vi "Begin.vi"(8 "error in":errorcluster) -> (0 "error out":errorcluster)   [LabVIEW 2023]
doc: "Called before other user functions, this VI is expected to open initial I/O refnums, load in file data, and do all program initialization. Notice that the <B>error out</B> terminal is simply used for data flow. Wiring it to other structures or subVIs ensures that this VI runs first."
uses:
  <vilib>/Rock Robotics/WPI/DriverStation/WPI_DriverStationRobotMode2.ctl
  <vilib>/Rock Robotics/WPI/Joystick/WPI_JoystickDeviceEnum.ctl
  <vilib>/Rock Robotics/WPI/SafetyOutput/WPI_SafetyOutputConfigMenu.ctl
  Robot Global Data.vi
  <vilib>/Rock Robotics/Network Tables/NT Write String Array.vi
  <vilib>/Rock Robotics/WPI/RobotDrive/WPI_RobotDriveOpen2MotorWithExistingMotors.vi
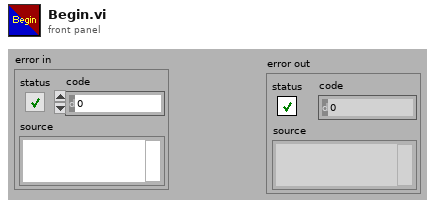
[diagram p1: front panel]
types:
  T1 = typedef "WPI_SafetyOutputConfigMenu.ctl" = enum16{"Enable", "Disable"}
  T2 = typedef "WPI_JoystickDeviceEnum.ctl" = enum16{"USB 0", "USB 1", "USB 2", "USB 3", "USB 4", "USB 5"}
  T3 = typedef "WPI_DriverStationRobotMode2.ctl" = enum16{"Autonomous Disabled", "Autonomous Enabled", "Teleop Disabled", "Teleop Enabled", "Disconnected", "Finish", "Test Disabled", "Test Enabled", "Emergency Stopped"}
  T4 = typedef "WPI_MotorControlDeviceRef.ctl" = cluster{"DeviceStatus":errorcluster, "Type":T5, "PWM":cluster{"PWM Channel":T6, "DeadBand":T7}, "CAN":cluster{"Device Number":u8, "SetOutput VI Ref":variant, "GetOutput VI Ref":variant, "Enable VI Ref":variant, "Disable VI Ref":variant, "Data":variant}, "Invert":bool, "DIO PWM":cluster{"PWM \"Enable\" Channel":T6, "DIOChannel":T8, "PWM Rate":dbl}}
  T5 = typedef "WPI_MotorControlType.ctl" = enum16{"PWM", "CAN", "DIO PWM"}
  T6 = typedef "FPGA_DIOPWMChannel.ctl" = enum8{"PWM 0", "PWM 1", "PWM 2", "PWM 3", "PWM 4", "PWM 5", "PWM 6", "PWM 7", "PWM 8", "PWM 9", "PWM MXP 0", "PWM MXP 1", "PWM MXP 2", "PWM MXP 3", "PWM MXP 4", "PWM MXP 5", "PWM MXP 6", "PWM MXP 7", "PWM MXP 8", "PWM MXP 9", "Invalid"}
  T7 = typedef "WPI_PWMDeadband.ctl" = cluster{"Name":string, "maxPositivePwm":i32, "minPositivePwm":i32, "centerPwm":i32, "maxNegativePwm":i32, "minNegativePwm":i32, "angularRange":u16}
  T8 = typedef "FPGA_DIOChannel.ctl" = enum8{"DIO 0", "DIO 1", "DIO 2", "DIO 3", "DIO 4", "DIO 5", "DIO 6", "DIO 7", "DIO 8", "DIO 9", "DIO MXP 0", "DIO MXP 1", "DIO MXP 2", "DIO MXP 3", "DIO MXP 4", "DIO MXP 5", "DIO MXP 6", "DIO MXP 7", "DIO MXP 8", "DIO MXP 9", "DIO MXP 10", "DIO MXP 11", "DIO MXP 12", "DIO MXP 13", "DIO MXP 14", "DIO MXP 15", "SPI Port CS1", "SPI Port CS2", "SPI Port CS3", "SPI Port MISO", "SPI Port MOSI", "Invalid"}
  T9 = typedef "WPI_RobotDriveDevRef.ctl" = cluster{"DevStatus":errorcluster, "Motors[]":T4[], "Square Inputs":bool, "Max Output":dbl}
  T10 = typedef "WPI_JoystickDevRef.ctl" = cluster{"Device":T2}
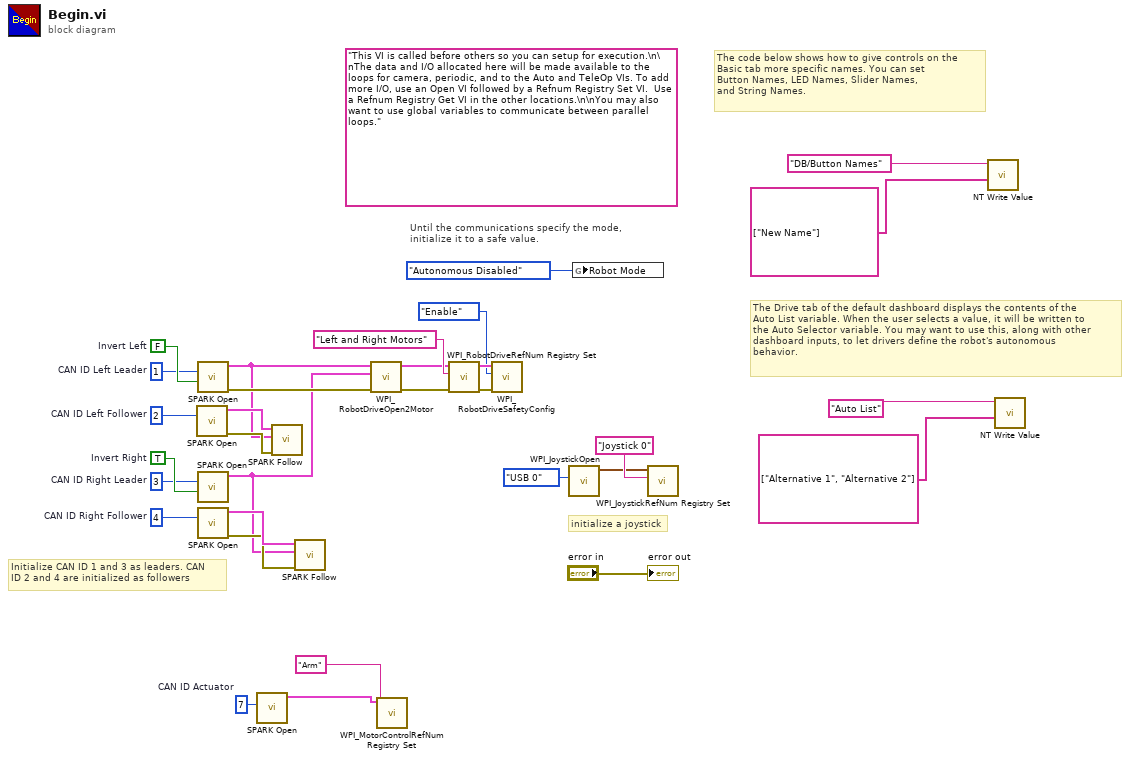
[diagram p0: block diagram]
diagram:
  w3 = u8 7  # CAN ID Actuator
  w22 = FALSE  # Invert Left
  w21 = TRUE  # Invert Right
  w13 = u8 3  # CAN ID Right Leader
  w14 = u8 4  # CAN ID Right Follower
  w6 = u8 1  # CAN ID Left Leader
  w5 = u8 2  # CAN ID Left Follower
  (unwired) "This VI is called before others so you can setup for execution.\n\nThe data and I/O allocated here will be made available to the loops for camera, periodic, and to the Auto and TeleOp VIs. To add more I/O, use an Open VI followed by a Refnum Registry Set VI.  Use a Refnum Registry Get VI in the other locations.\n\nYou may also want to use global variables to communicate between parallel loops."
  # "Initialize CAN ID 1 and 3 as leaders. CAN \nID 2 and 4 are initialized as followers"
  # "The Drive tab of the default dashboard displays the contents of the\nAuto List variable. When the user selects a value, it will be written to\nthe Auto Selector variable. You may want to use this, along with other\ndashboard inputs, to let drivers define the robot's autonomous\nbehavior."
  # "The code below shows how to give controls on the\nBasic tab more specific names. You can set\nButton Names, LED Names, Slider Names,\nand String Names."
  # "initialize a joystick"
  # "Until the communications specify the mode,\ninitialize it to a safe value."
  n1 = call <vilib>:"SPARK Open.vi"("Device Number"=w5) -> ("error out"=w10:errorcluster, "MotorControlDeviceRef"=w9:T4)  [unwired: 9 in]
  n2 = call <vilib>:"SPARK Open.vi"("Invert"=w22, "Device Number"=w6) -> ("error out"=w8:errorcluster, "MotorControlDeviceRef"=w7:T4)  [unwired: 8 in]
  n3 = call <vilib>:"SPARK Open.vi"("Invert"=w21, "Device Number"=w13) -> ("MotorControlDeviceRef"=w4:T4)  [unwired: 8 in, 1 out]
  n4 = call <vilib>:"SPARK Open.vi"("Device Number"=w14) -> ("error out"=w11:errorcluster, "MotorControlDeviceRef"=w12:T4)  [unwired: 9 in]
  n5 = call <vilib>:"SPARK Open.vi"("Device Number"=w3) -> ("MotorControlDeviceRef"=w2:T4)  [unwired: 9 in, 1 out]
  n6 = call <vilib>:"SPARK Follow.vi"("error in (no error)"=w10, "Master Controller"=w7, "MotorControlDeviceRef"=w9) -> ()  [unwired: 7 in, 2 out]
  n7 = call <vilib>:"SPARK Follow.vi"("error in (no error)"=w11, "Master Controller"=w4, "MotorControlDeviceRef"=w12) -> ()  [unwired: 7 in, 2 out]
  n8 = call-poly <vilib>:"WPI_RobotDriveOpen2Motor.vi"("error in (no error)"=w8, "Right Motor Dev Ref"=w4, "Left Motor Dev Ref"=w7) -> ("error out"=w17:errorcluster, "RobotDriveDevRef"=w15:T9)  [unwired: 7 in]
  n9 = call <vilib>:"WPI_MotorControlRefNum Registry Set.vi"("refnum name"="Arm", "MotorControlDevRef"=w2) -> ()  [unwired: 8 in, 2 out]
  n10 = call <vilib>:"WPI_RobotDriveRefNum Registry Set.vi"("error in (no error)"=w17, "refnum name"="Left and Right Motors", "RobotDriveDevRef"=w15) -> ("error out"=w20:errorcluster, "RobotDriveDevRef"=w19:T9)  [unwired: 7 in]
  n11 = call <vilib>:"WPI_RobotDriveSafetyConfig.vi"("error in (no error)"=w20, "mode"=WPI_SafetyOutputConfigMenu."Enable", "RobotDriveDevRef"=w19) -> ()  [unwired: 7 in, 2 out]
  n12 = call <vilib>:"WPI_JoystickOpen.vi"("JoystickDevice"=WPI_JoystickDeviceEnum."USB 0") -> ("JoystickDevRef"=w29:T10)  [unwired: 10 in]
  n13 = global write "Robot Global Data.vi" "Robot Mode"(WPI_DriverStationRobotMode2."Autonomous Disabled" ("Robot Mode")) -> ()
  n14 = call <vilib>:"WPI_JoystickRefNum Registry Set.vi"("refnum name"="Joystick 0", "JoystickDevRef"=w29) -> ()  [unwired: 8 in, 2 out]
  n15 = call-poly <vilib>:"NT Write Value.vi"("value"=string[] ["New Name"], "name"="DB/Button Names" ("Name")) -> ()  [unwired: 9 in, 1 out]
  n16 = call-poly <vilib>:"NT Write Value.vi"("value"=string[] ["Alternative 1", "Alternative 2"] ("String Array"), "name"="Auto List" ("Name")) -> ()  [unwired: 9 in, 1 out]
  "error out" <- "error in"
